vi "get voltage range ring.vi"(8 "error in (no error)":errorcluster caption="에러 입력(에러 없음)", 11 "DW7802 입력":refnum<class "DW7802.lvclass">) -> (0 "error out":errorcluster caption="에러 출력", 1 "caption":string="VD Clamp", 2 "strings & values":T1=[{"String"="0.000V", "Value"=0.0}, {"String"="0.024V", "Value"=0.024}, {"String"="0.048V", "Value"=0.048}, {"String"="0.072V", "Value"=0.072}, {"String"="0.096V", "Value"=0.096}, {"String"="0.120V", "Value"=0.12}, {"String"="0.144V", "Value"=0.144}, {"String"="0.168V", "Value"=0.168}, {"String"="0.192V", "Value"=0.192}, {"String"="0.216V", "Value"=0.216}, {"String"="0.240V", "Value"=0.24}, {"String"="0.264V", "Value"=0.264}, {"String"="0.288V", "Value"=0.288}, {"String"="0.312V", "Value"=0.312}, {"String"="0.336V", "Value"=0.336}, {"String"="0.360V", "Value"=0.36}, {"String"="0.384V", "Value"=0.384}, {"String"="0.408V", "Value"=0.408}, {"String"="0.432V", "Value"=0.432}, {"String"="0.456V", "Value"=0.456}, {"String"="0.480V", "Value"=0.48}, {"String"="0.504V", "Value"=0.504}, {"String"="0.528V", "Value"=0.528}, {"String"="0.552V", "Value"=0.552}, {"String"="0.576V", "Value"=0.576}, {"String"="0.600V", "Value"=0.6}, {"String"="0.624V", "Value"=0.624}, {"String"="0.648V", "Value"=0.648}, {"String"="0.672V", "Value"=0.672}, {"String"="0.696V", "Value"=0.696}, {"String"="0.720V", "Value"=0.72}, {"String"="0.744V", "Value"=0.744}, {"String"="0.768V", "Value"=0.768}, {"String"="0.792V", "Value"=0.792}, {"String"="0.816V", "Value"=0.816}, {"String"="0.840V", "Value"=0.84}, {"String"="0.864V", "Value"=0.864}, {"String"="0.888V", "Value"=0.888}, {"String"="0.912V", "Value"=0.912}, {"String"="0.936V", "Value"=0.936}, {"String"="0.960V", "Value"=0.96}, {"String"="0.984V", "Value"=0.984}, {"String"="1.008V", "Value"=1.008}, {"String"="1.032V", "Value"=1.032}, {"String"="1.056V", "Value"=1.056}, {"String"="1.080V", "Value"=1.08}, {"String"="1.104V", "Value"=1.104}, {"String"="1.128V", "Value"=1.128}, {"String"="1.152V", "Value"=1.152}, {"String"="1.176V", "Value"=1.176}, {"String"="1.200V", "Value"=1.2}, {"String"="1.224V", "Value"=1.224}, {"String"="1.248V", "Value"=1.248}, {"String"="1.272V", "Value"=1.272}, {"String"="1.296V", "Value"=1.296}, {"String"="1.320V", "Value"=1.32}, {"String"="1.344V", "Value"=1.344}, {"String"="1.368V", "Value"=1.368}, {"String"="1.392V", "Value"=1.392}, {"String"="1.416V", "Value"=1.416}, {"String"="1.440V", "Value"=1.44}, {"String"="1.464V", "Value"=1.464}, {"String"="1.488V", "Value"=1.488}, {"String"="1.512V", "Value"=1.512}, {"String"="1.536V", "Value"=1.536}, {"String"="1.560V", "Value"=1.56}, {"String"="1.584V", "Value"=1.584}, {"String"="1.608V", "Value"=1.608}, {"String"="1.632V", "Value"=1.632}, {"String"="1.656V", "Value"=1.656}, {"String"="1.680V", "Value"=1.68}, {"String"="1.704V", "Value"=1.704}, {"String"="1.728V", "Value"=1.728}, {"String"="1.752V", "Value"=1.752}, {"String"="1.776V", "Value"=1.776}, {"String"="1.800V", "Value"=1.8}, {"String"="1.824V", "Value"=1.824}, {"String"="1.848V", "Value"=1.848}, {"String"="1.872V", "Value"=1.872}, {"String"="1.896V", "Value"=1.896}, {"String"="1.920V", "Value"=1.92}, {"String"="1.944V", "Value"=1.944}, {"String"="1.968V", "Value"=1.968}, {"String"="1.992V", "Value"=1.992}, {"String"="2.016V", "Value"=2.016}, {"String"="2.040V", "Value"=2.04}, {"String"="2.064V", "Value"=2.064}, {"String"="2.088V", "Value"=2.088}, {"String"="2.112V", "Value"=2.112}, {"String"="2.136V", "Value"=2.136}, {"String"="2.160V", "Value"=2.16}, {"String"="2.184V", "Value"=2.184}, {"String"="2.208V", "Value"=2.208}, {"String"="2.232V", "Value"=2.232}, {"String"="2.256V", "Value"=2.256}, {"String"="2.280V", "Value"=2.28}, {"String"="2.304V", "Value"=2.304}, {"String"="2.328V", "Value"=2.328}, {"String"="2.352V", "Value"=2.352}, {"String"="2.376V", "Value"=2.376}, {"String"="2.400V", "Value"=2.4}, {"String"="2.424V", "Value"=2.424}, {"String"="2.448V", "Value"=2.448}, {"String"="2.472V", "Value"=2.472}, {"String"="2.496V", "Value"=2.496}, {"String"="2.520V", "Value"=2.52}, {"String"="2.544V", "Value"=2.544}, {"String"="2.568V", "Value"=2.568}, {"String"="2.592V", "Value"=2.592}, {"String"="2.616V", "Value"=2.616}, {"String"="2.640V", "Value"=2.64}, {"String"="2.664V", "Value"=2.664}, {"String"="2.688V", "Value"=2.688}, {"String"="2.712V", "Value"=2.712}, {"String"="2.736V", "Value"=2.736}, {"String"="2.760V", "Value"=2.76}, {"String"="2.784V", "Value"=2.784}, {"String"="2.808V", "Value"=2.808}, {"String"="2.832V", "Value"=2.832}, {"String"="2.856V", "Value"=2.856}, {"String"="2.880V", "Value"=2.88}, {"String"="2.904V", "Value"=2.904}, {"String"="2.928V", "Value"=2.928}, {"String"="2.952V", "Value"=2.952}, {"String"="2.976V", "Value"=2.976}, {"String"="3.000V", "Value"=3.0}, {"String"="3.024V", "Value"=3.024}, {"String"="3.048V", "Value"=3.048}, {"String"="3.072V", "Value"=3.072}, {"String"="3.096V", "Value"=3.096}, {"String"="3.120V", "Value"=3.12}, {"String"="3.144V", "Value"=3.144}, {"String"="3.168V", "Value"=3.168}, {"String"="3.192V", "Value"=3.192}, {"String"="3.216V", "Value"=3.216}, {"String"="3.240V", "Value"=3.24}, {"String"="3.264V", "Value"=3.264}, {"String"="3.288V", "Value"=3.288}, {"String"="3.312V", "Value"=3.312}, {"String"="3.336V", "Value"=3.336}, {"String"="3.360V", "Value"=3.36}, {"String"="3.384V", "Value"=3.384}, {"String"="3.408V", "Value"=3.408}, {"String"="3.432V", "Value"=3.432}, {"String"="3.456V", "Value"=3.456}, {"String"="3.480V", "Value"=3.48}, {"String"="3.504V", "Value"=3.504}, {"String"="3.528V", "Value"=3.528}, {"String"="3.552V", "Value"=3.552}, {"String"="3.576V", "Value"=3.576}, {"String"="3.600V", "Value"=3.6}, {"String"="3.624V", "Value"=3.624}, {"String"="3.648V", "Value"=3.648}, {"String"="3.672V", "Value"=3.672}, {"String"="3.696V", "Value"=3.696}, {"String"="3.720V", "Value"=3.72}, {"String"="3.744V", "Value"=3.744}, {"String"="3.768V", "Value"=3.768}, {"String"="3.792V", "Value"=3.792}, {"String"="3.816V", "Value"=3.816}, {"String"="3.840V", "Value"=3.84}, {"String"="3.864V", "Value"=3.864}, {"String"="3.888V", "Value"=3.888}, {"String"="3.912V", "Value"=3.912}, {"String"="3.936V", "Value"=3.936}, {"String"="3.960V", "Value"=3.96}, {"String"="3.984V", "Value"=3.984}, {"String"="4.008V", "Value"=4.008}, {"String"="4.032V", "Value"=4.032}, {"String"="4.056V", "Value"=4.056}, {"String"="4.080V", "Value"=4.08}, {"String"="4.104V", "Value"=4.104}, {"String"="4.128V", "Value"=4.128}, {"String"="4.152V", "Value"=4.152}, {"String"="4.176V", "Value"=4.176}, {"String"="4.200V", "Value"=4.2}, {"String"="4.224V", "Value"=4.224}, {"String"="4.248V", "Value"=4.248}, {"String"="4.272V", "Value"=4.272}, {"String"="4.296V", "Value"=4.296}, {"String"="4.320V", "Value"=4.32}, {"String"="4.344V", "Value"=4.344}, {"String"="4.368V", "Value"=4.368}, {"String"="4.392V", "Value"=4.392}, {"String"="4.416V", "Value"=4.416}, {"String"="4.440V", "Value"=4.44}, {"String"="4.464V", "Value"=4.464}, {"String"="4.488V", "Value"=4.488}, {"String"="4.512V", "Value"=4.512}, {"String"="4.536V", "Value"=4.536}, {"String"="4.560V", "Value"=4.56}, {"String"="4.584V", "Value"=4.584}, {"String"="4.608V", "Value"=4.608}, {"String"="4.632V", "Value"=4.632}, {"String"="4.656V", "Value"=4.656}, {"String"="4.680V", "Value"=4.68}, {"String"="4.704V", "Value"=4.704}, {"String"="4.728V", "Value"=4.728}, {"String"="4.752V", "Value"=4.752}, {"String"="4.776V", "Value"=4.776}, {"String"="4.800V", "Value"=4.8}, {"String"="4.824V", "Value"=4.824}, {"String"="4.848V", "Value"=4.848}, {"String"="4.872V", "Value"=4.872}, {"String"="4.896V", "Value"=4.896}, {"String"="4.920V", "Value"=4.92}, {"String"="4.944V", "Value"=4.944}, {"String"="4.968V", "Value"=4.968}, {"String"="4.992V", "Value"=4.992}, {"String"="5.016V", "Value"=5.016}, {"String"="5.040V", "Value"=5.04}, {"String"="5.064V", "Value"=5.064}, {"String"="5.088V", "Value"=5.088}, {"String"="5.112V", "Value"=5.112}, {"String"="5.136V", "Value"=5.136}, {"String"="5.160V", "Value"=5.16}, {"String"="5.184V", "Value"=5.184}, {"String"="5.208V", "Value"=5.208}, {"String"="5.232V", "Value"=5.232}, {"String"="5.256V", "Value"=5.256}, {"String"="5.280V", "Value"=5.28}, {"String"="5.304V", "Value"=5.304}, {"String"="5.328V", "Value"=5.328}, {"String"="5.352V", "Value"=5.352}, {"String"="5.376V", "Value"=5.376}, {"String"="5.400V", "Value"=5.4}, {"String"="5.424V", "Value"=5.424}, {"String"="5.448V", "Value"=5.448}, {"String"="5.472V", "Value"=5.472}, {"String"="5.496V", "Value"=5.496}, {"String"="5.520V", "Value"=5.52}, {"String"="5.544V", "Value"=5.544}, {"String"="5.568V", "Value"=5.568}, {"String"="5.592V", "Value"=5.592}, {"String"="5.616V", "Value"=5.616}, {"String"="5.640V", "Value"=5.64}, {"String"="5.664V", "Value"=5.664}, {"String"="5.688V", "Value"=5.688}, {"String"="5.712V", "Value"=5.712}, {"String"="5.736V", "Value"=5.736}, {"String"="5.760V", "Value"=5.76}, {"String"="5.784V", "Value"=5.784}, {"String"="5.808V", "Value"=5.808}, {"String"="5.832V", "Value"=5.832}, {"String"="5.856V", "Value"=5.856}, {"String"="5.880V", "Value"=5.88}, {"String"="5.904V", "Value"=5.904}, {"String"="5.928V", "Value"=5.928}, {"String"="5.952V", "Value"=5.952}, {"String"="5.976V", "Value"=5.976}, {"String"="6.000V", "Value"=6.0}, {"String"="6.024V", "Value"=6.024}, {"String"="6.048V", "Value"=6.048}, {"String"="6.072V", "Value"=6.072}, {"String"="6.096V", "Value"=6.096}, {"String"="6.120V", "Value"=6.12}], 3 "DW7802 출력":refnum<class "DW7802.lvclass">, 4 "read value":dbl=2.04)   [LabVIEW 2020, in "DW7802.lvclass"]
uses:
  DW7802.lvclass
  <vilib>/Utility/miscctls.llb/LVStringsAndValuesArrayTypeDef_DBL.ctl
  Haptic IC/Haptic IC.lvclass/Haptic IC.ctl
  SubVIs/I2C/Instance VIs/(SubVI)I2C_8Bit-8Bit_Read_Single.vi
  Haptic IC/Haptic IC.lvclass
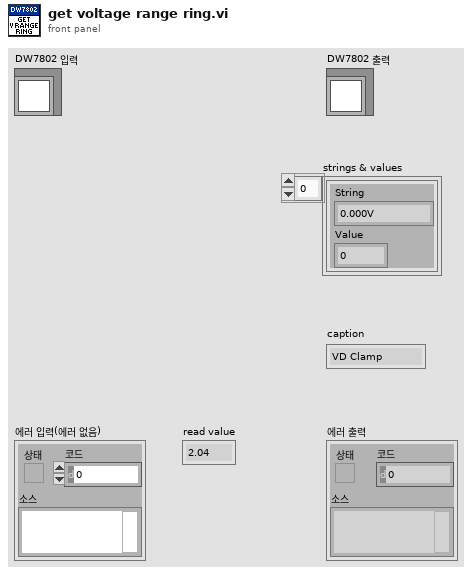
[diagram p1: front panel]
types:
  T1 = typedef "LVStringsAndValuesArrayTypeDef_DBL.ctl" = cluster{"String":string, "Value":dbl}[]
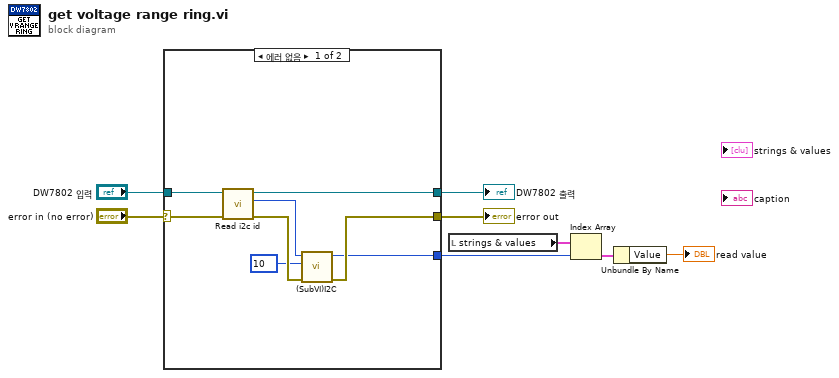
[diagram p0: block diagram]
diagram:
  n1 = case shown="에러 없음" "error in (no error)" {
    selector: "error in (no error)" -> [w16 w18]
    tunnel: [w15 w17] -> w5
    tunnel: [w11 w18] -> w4
    tunnel: [w10 _] -> w8
    tunnel: "DW7802 입력" -> [w9 w17]
    frame No Error {
      n2 = call "Read i2c id.vi"("error in (no error)"=w16, "Haptic IC 입력"=w9) -> ("error out"=w14:errorcluster, "i2c id"=w13:u8, "Haptic IC 출력"=w15:refnum<class "DW7802.lvclass">)  [unwired: 7 in]
      n3 = call-poly "(SubVI)I2C.vi"("error in (no error)"=w14, "Address"=u8 10, "ID"=w13) -> ("error out"=w11:errorcluster, "Read Data"=w10:u8)  [unwired: 6 in, 1 out]
    }
    frame Error {
    }
  }
  "error out" <- w4
  "DW7802 출력" <- w5
  n4 = local read "strings & values"() -> (w3:T1)
  n5 = Index Array(array=w3, index=w8) -> (element=w2:cluster{"String":string, "Value":dbl})
  n6 = Unbundle By Name(w2) -> ("Value"=→"read value":dbl)
